vi "reservoir 1.vi"() -> ()   [LabVIEW 2018]
panel:
  in  "stop":bool
  out "Tank":i32(slide) scale=0.0..1100.0
  in  "Débit":u8(slide) scale=0.0..10.0
  in  "Consigne":i32(slide) scale=0.0..1000.0
  out "valeur tank":u8
  in  "valeur consigne":u8
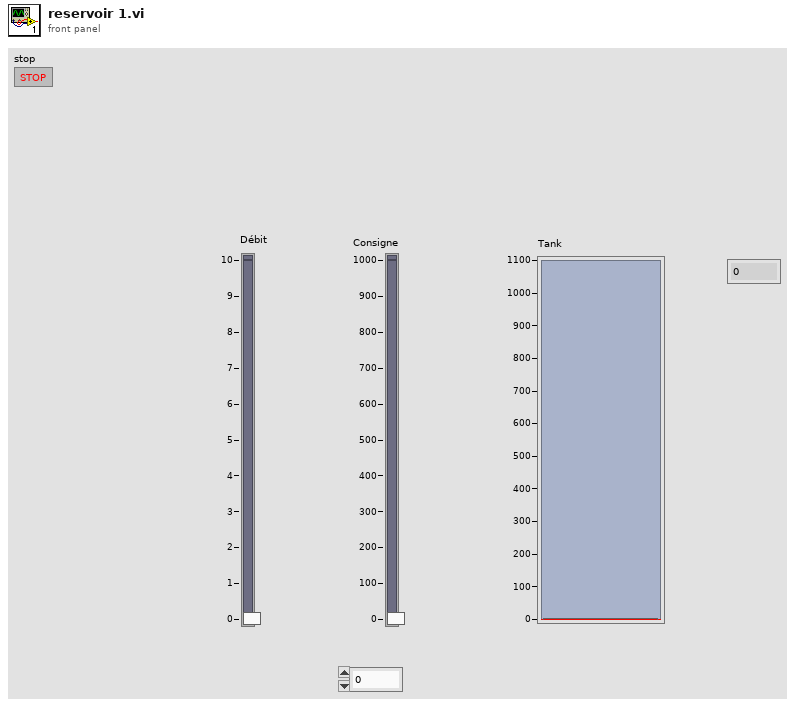
[diagram p1: front panel]
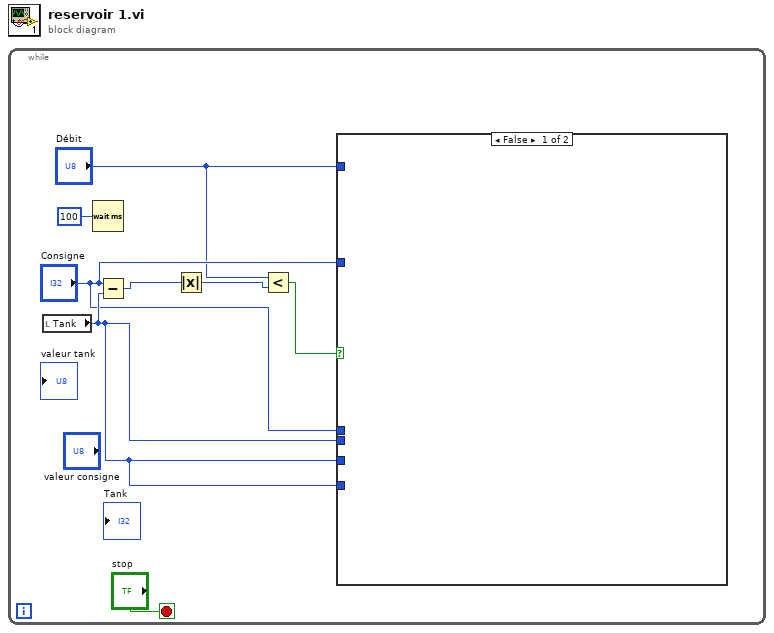
[diagram p0: block diagram]
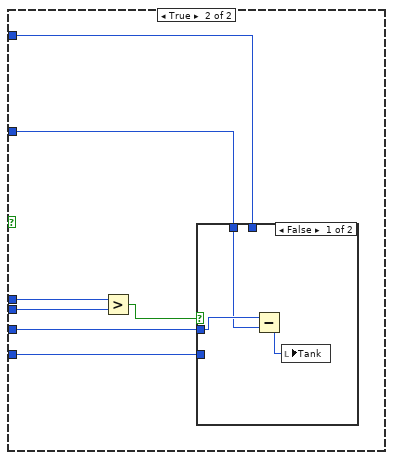
[diagram p2: hidden frame]
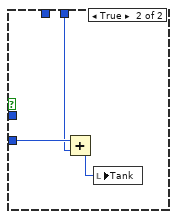
[diagram p3: hidden frame]
diagram:
  n1 = while {
    stop <- "stop" stop-if-true
    n2 = local read "Tank"() -> (w4:i32)
    n3 = Wait (ms)(milliseconds to wait=u32 100) -> ()  [unwired: 1 out]
    n4 = Subtract(x="Consigne", y=w4) -> (x-y=w6:i32)
    n5 = Absolute Value(x=w6) -> (abs(x)=w1:i32)
    n6 = Less?(x="Débit", y=w1) -> (x < y?=w5:bool)
    n7 = case shown="False" w5 {
      tunnel: "Consigne" -> [_ w15]
      tunnel: w4 -> [_ w14]
      tunnel: w4 -> [_ w12]
      tunnel: "Débit" -> [_ w11]
      tunnel: w4 -> [_ w10]
      tunnel: "Consigne" -> [_ w9]
      frame False {
      }
      frame True {
        n8 = Greater?(x=w15, y=w14) -> (0:w13:bool)
        n9 = case shown="False" w13 {
          tunnel: w12 -> [_ w21]
          tunnel: w11 -> [_ w20]
          tunnel: w10 -> [w18 _]
          tunnel: w9 -> [w17 _]
          frame False {
            n10 = Subtract(x=w18, y=w17) -> (x-y=w16:i32)
            n11 = local write "Tank"(w16) -> ()
          }
          frame True {
            n12 = Add(x=w21, y=w20) -> (x+y=w19:i32)
            n13 = local write "Tank"(w19) -> ()
          }
        }
      }
    }
  }
